vi "Finish Recording.vi"(8 "error in (no error)":errorcluster, 11 "Application in":refnum<class "Application.lvclass">) -> (0 "error out":errorcluster, 3 "Application out":refnum<class "Application.lvclass">)   [LabVIEW 2023, in "Application.lvlib" / "Application.lvclass"]
uses:
  Application.lvclass
  Mode.ctl
  Application.lvclass/Application.ctl
  User Interface/Main Window Messages/Application Mode Change Msg/Application Mode Change Msg.lvclass/Application Mode Change Msg.ctl
  <vilib>/ActorFramework/Message Enqueuer/Message Enqueuer.lvclass/Message Enqueuer.ctl
  <vilib>/ActorFramework/Message Enqueuer/Enqueue.vi
  User Interface/Main Window Messages/Application Mode Change Msg/Application Mode Change Msg.lvclass
  C:/Program Files/National Instruments/LabVIEW 2023/vi.lib/ActorFramework/Message/Message.lvclass
  <vilib>/ActorFramework/Message Priority Queue/Priority Enqueue.vi
  Application.lvlib
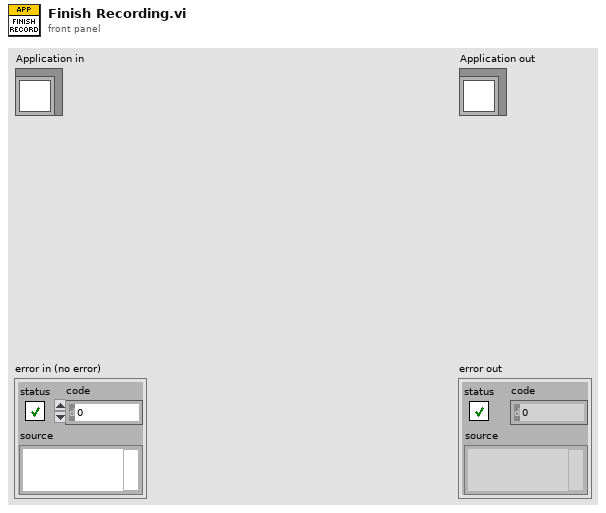
[diagram p1: front panel]
types:
  T1 = typedef "Application.lvlib/Mode.ctl" = enum16{"Idle", "Cancel", "Live", "Stream", "Autofocus", "Z-Stack"}
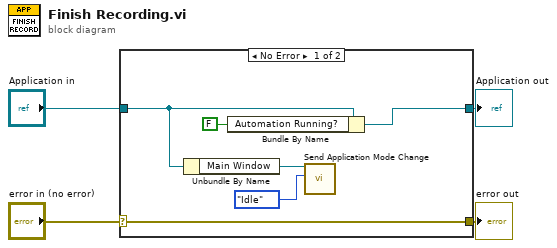
[diagram p0: block diagram]
diagram:
  n1 = case shown="No Error" "error in (no error)" {
    selector: "error in (no error)" -> [w10 w12]
    tunnel: [w10 w12] -> w3
    tunnel: [w9 w11] -> w1
    tunnel: "Application in" -> [w7 w11]
    frame No Error {
      n2 = Unbundle By Name(w7) -> ("Main Window"=w6:refnum<class "Message Enqueuer.lvclass">)
      n3 = Bundle By Name(cluster=w7, "Automation Running?"=FALSE) -> (w9:refnum<class "Application.lvclass">)
      n4 = call "Send Application Mode Change.vi"("Mode"=Mode."Idle", "Message Enqueuer"=w6) -> ()  [unwired: 8 in, 2 out]
    }
    frame Error {
    }
  }
  "error out" <- w3
  "Application out" <- w1
